vi "Main.vi"() -> ()   [LabVIEW 2020]
uses:
  <vilib>/Utility/config.llb/Read Key (String).vi
  <vilib>/Utility/file.llb/Write Delimited Spreadsheet (string).vi
  <vilib>/Utility/config.llb/NI_LVConfig.lvlib
panel:
  out "状态显示":bool=TRUE
  in  "开始测试":bool
  out "绝缘电阻采样测试":T1={"正极绝缘电阻"=0.0, "负极绝缘电阻"=0.0, "总判定"=TRUE}
  out "电流校准测试结果":T2={"表格控件"=[], "斜率"=0.0, "截距"=0.0, "判定"=TRUE}
  out "导通电阻":T3={"阻值"={"主保险"=0.0, "主正继电器"=0.0, "快充继电器"=0.0, "主负继电器"=0.0, "分流器"=0.0}, "判定"={"布尔"=TRUE, "布尔 2"=TRUE, "布尔 3"=TRUE, "布尔 4"=TRUE, "布尔 5"=TRUE}}
  out "Vact判定":bool=TRUE
  out "表格控件":string[][](table) caption="电压采样精度检测"
  out "短接快充":T4={"簇"={"Va"=0, "Vc"=0, "Vd"=0, "Vg"=0}, "判定"={"判定"=TRUE, "判定"=TRUE, "判定"=TRUE, "判定"=TRUE}}
  out "闭合主正快充":T4={"簇"={"Va"=0, "Vc"=0, "Vd"=0, "Vg"=0}, "判定"={"判定"=TRUE, "判定"=TRUE, "判定"=TRUE, "判定"=TRUE}}
  out "闭合主正":T4={"簇"={"Va"=0, "Vc"=0, "Vd"=0, "Vg"=0}, "判定"={"判定"=TRUE, "判定"=TRUE, "判定"=TRUE, "判定"=TRUE}}
  out "全部打开":T4={"簇"={"Va"=0, "Vc"=0, "Vd"=0, "Vg"=0}, "判定"={"判定"=TRUE, "判定"=TRUE, "判定"=TRUE, "判定"=TRUE}}
  out "预充电阻":dbl
  out "通断检测":T5={"粘连检测"={TRUE, TRUE, TRUE}, "导通检测"={"主保险"=0.0, "主正继电器"=0.0, "主负继电器"=0.0, "快充继电器"=0.0}, "簇"={TRUE, TRUE, TRUE, TRUE}}
  out "HVIL":T7={"占空比"=0, "频率/周期"=0, "软件版本号"=0, "频率判定"=TRUE, "占空比判定"=TRUE, "软件版本指示"=0} {"软件版本指示" items=["for 广汽新能源"=24015, "for 中航锂电"=25018]}
  out "CMC":cluster{"表格控件":string[][], "啊打发":bool}={"表格控件"=[], "啊打发"=TRUE}
  in  "停止":bool
  in  "value":string caption="序列号"
  # "F020电性能测试"
  # "47~53Ω"
  # "240~360kΩ"
  # "400~600kΩ"
  # "≤0.3"
  # "≤0.5"
  # "≤0.5"
  # "≤0.5"
  # "≤0.15"
  # "主正&预充"
  # "主负"
  # "快充"
  # "HVIL测试"
  # "Hz"
  # "判定：7~11Hz"
  # "判定：50±4%"
  # "%"
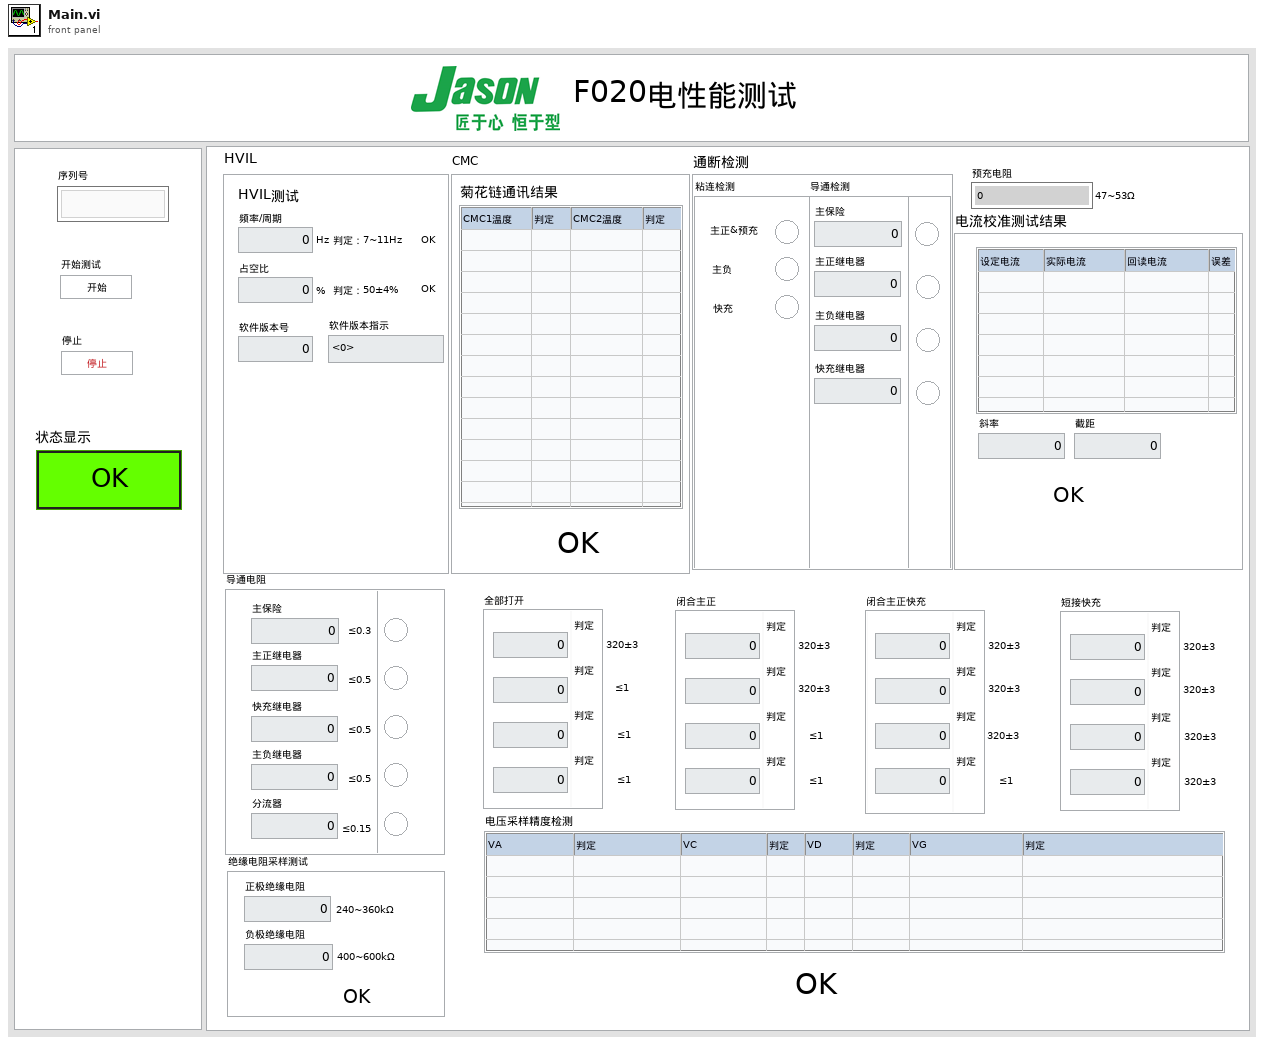
[diagram p1: front panel]
types:
  T1 = typedef "绝缘电阻测试.ctl" = cluster{"正极绝缘电阻":dbl, "负极绝缘电阻":dbl, "总判定":bool}
  T2 = typedef "电流校准测试.ctl" = cluster{"表格控件":string[][], "斜率":dbl, "截距":dbl, "判定":bool}
  T3 = typedef "导通电阻.ctl" = cluster{"阻值":cluster{"主保险":dbl, "主正继电器":dbl, "快充继电器":dbl, "主负继电器":dbl, "分流器":dbl}, "判定":cluster{"布尔":bool, "布尔 2":bool, "布尔 3":bool, "布尔 4":bool, "布尔 5":bool}}
  T4 = typedef "闭合主正.ctl" = cluster{"簇":cluster{"Va":u32, "Vc":u32, "Vd":u32, "Vg":u32}, "判定":cluster{"判定":bool, "判定":bool, "判定":bool, "判定":bool}}
  T5 = typedef "导通.ctl" = cluster{"粘连检测":cluster{bool, bool, bool}, "导通检测":cluster{"主保险":dbl, "主正继电器":dbl, "主负继电器":dbl, "快充继电器":dbl}, "簇":cluster{bool, bool, bool, bool}}
  T6 = typedef "软件版本指示.ctl" = u32
  T7 = cluster{"占空比":u32, "频率/周期":u32, "软件版本号":u32, "频率判定":bool, "占空比判定":bool, "软件版本指示":T6}
  T8 = typedef "状态机.ctl" = enum16{"Idle", "power on", "comm test", "conduct test", "resistance test", "Vact test", "insl test", "curr cal", "power off", "data log", "exit"}
  T9 = typedef "仪器地址输入.ctl" = cluster{"[0]":string, "[PLC]":string, "[IT6332B-1]":string, "[IT6332B-2]":string, "[2700-1]":string, "[2700-2]":string, "[TDK]":string, "[2410]":string}
  T10 = typedef "仪器实例.ctl" = cluster{"[0]":string, "[PLC]":refnum<k24>, "[IT6332B-1]":string, "[IT6332B-2]":string, "[2700-1]":string, "[2700-2]":string, "[TDK]":string, "[2410]":string}
  T11 = typedef "NI_LVConfig.lvlib/Config Data RefNum.ctl" = refnum<k1>
  T12 = cluster{"粘连判断[0]":bool, "粘连判断[1]":bool, "粘连判断[2]":bool}
  T13 = cluster{"导通值[0]":dbl, "导通值[1]":dbl, "导通值[2]":dbl, "导通值[3]":dbl}
  T14 = cluster{"导通判断[0]":bool, "导通判断[1]":bool, "导通判断[2]":bool, "导通判断[3]":bool}
  T15 = cluster{"导通电阻[0]":dbl, "导通电阻[1]":dbl, "导通电阻[2]":dbl, "导通电阻[3]":dbl, "导通电阻[4]":dbl}
  T16 = cluster{"x <= y?[0]":bool, "x <= y?[1]":bool, "x <= y?[2]":bool, "x <= y?[3]":bool, "x <= y?[4]":bool}
  T17 = cluster{"导通电阻":cluster{"导通电阻[0]":dbl, "导通电阻[1]":dbl, "导通电阻[2]":dbl, "导通电阻[3]":dbl, "导通电阻[4]":dbl}, "x <= y?":cluster{"x <= y?[0]":bool, "x <= y?[1]":bool, "x <= y?[2]":bool, "x <= y?[3]":bool, "x <= y?[4]":bool}}
  T18 = cluster{"布尔":bool, "布尔 2":bool, "布尔 3":bool, "布尔 4":bool, "布尔 5":bool}
  T19 = cluster{"主保险":dbl, "主正继电器":dbl, "快充继电器":dbl, "主负继电器":dbl, "分流器":dbl}
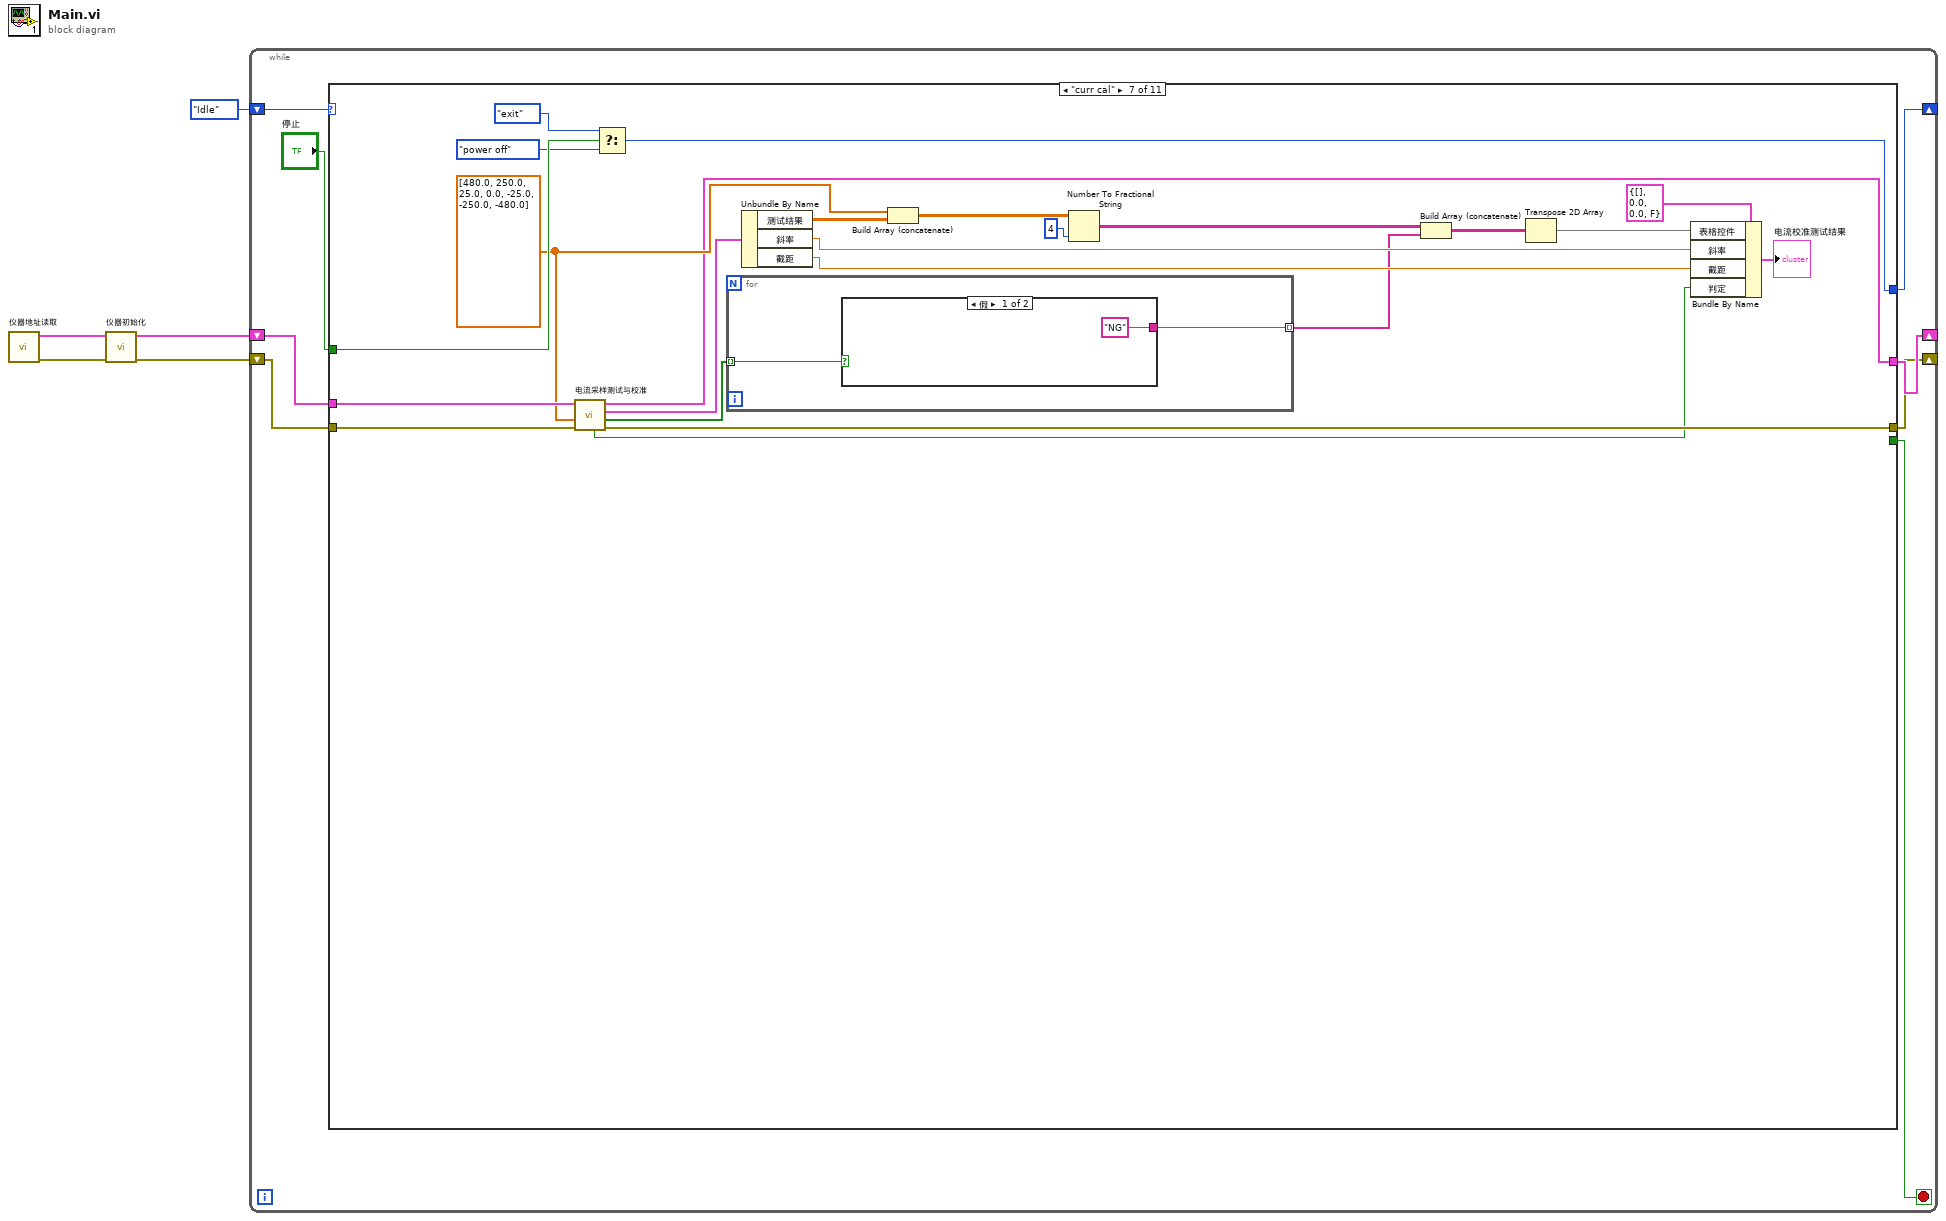
[diagram p0: block diagram]
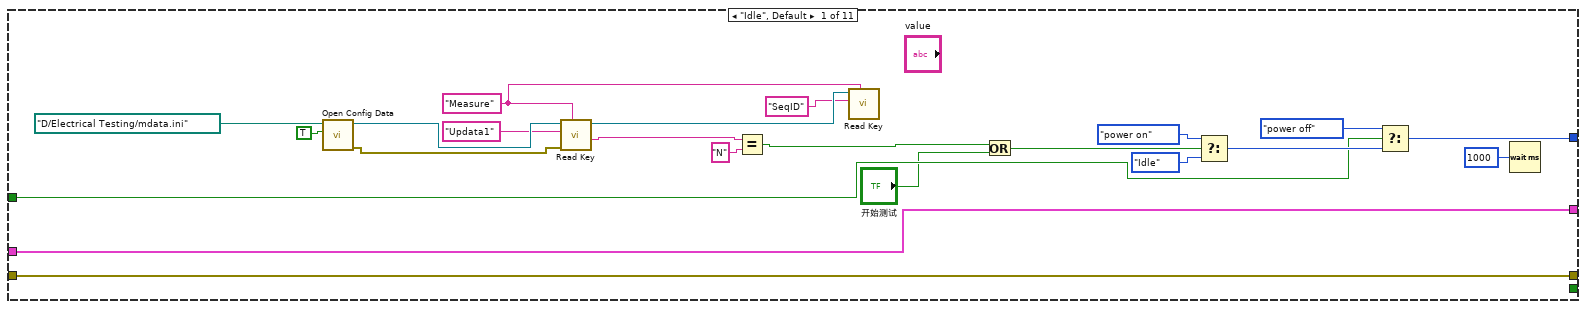
[diagram p2: hidden frame]
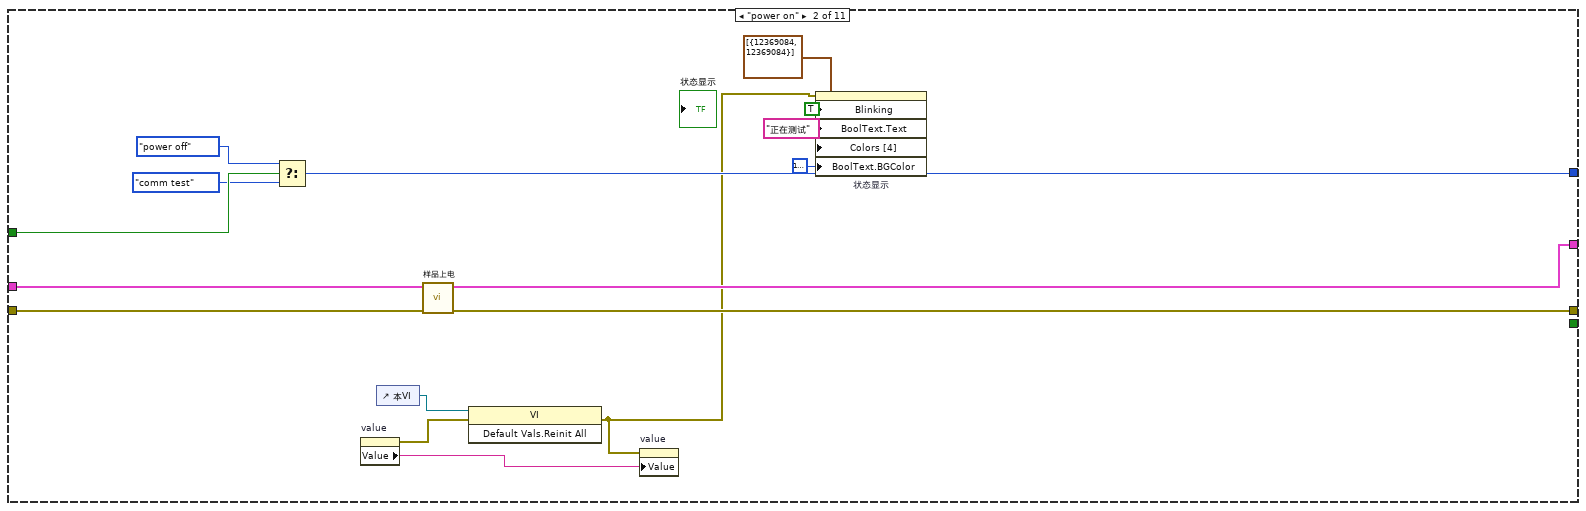
[diagram p3: hidden frame]
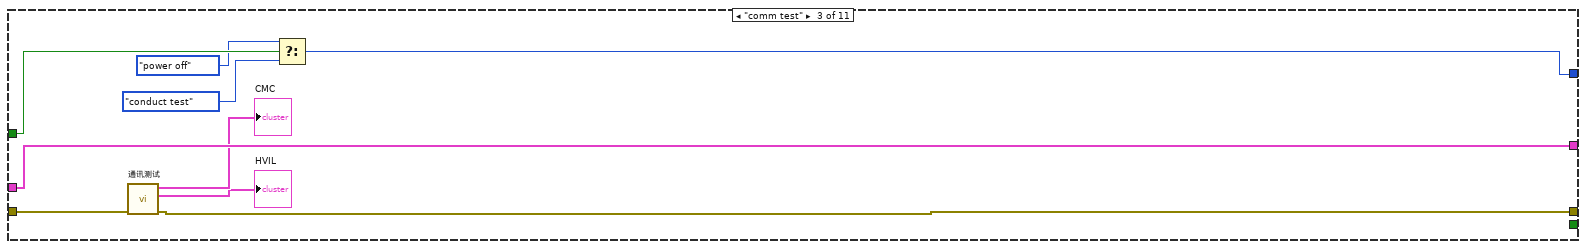
[diagram p4: hidden frame]
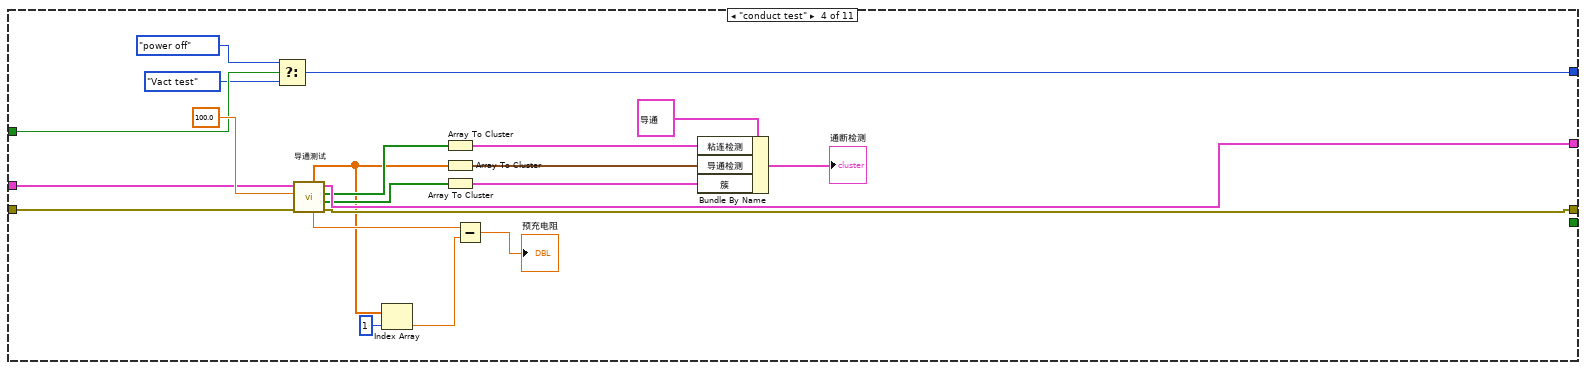
[diagram p5: hidden frame]
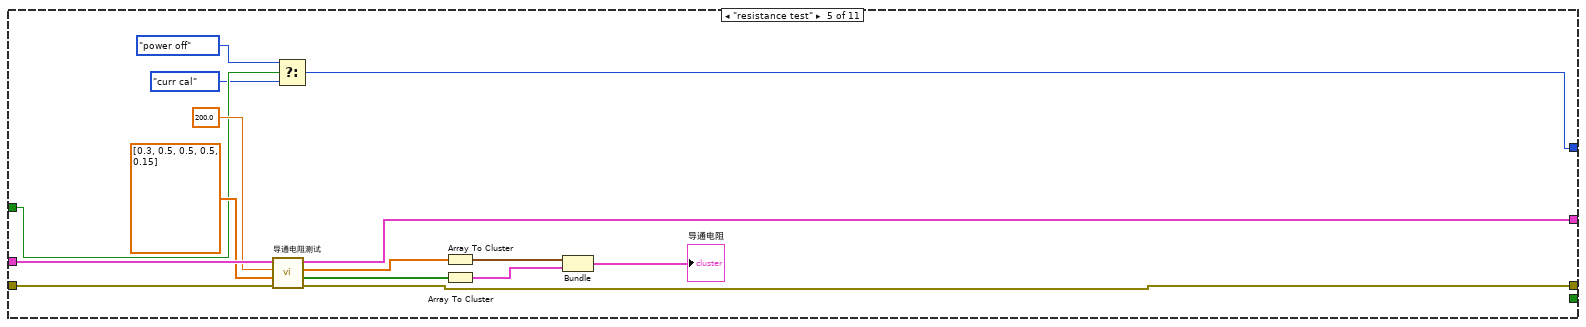
[diagram p6: hidden frame]
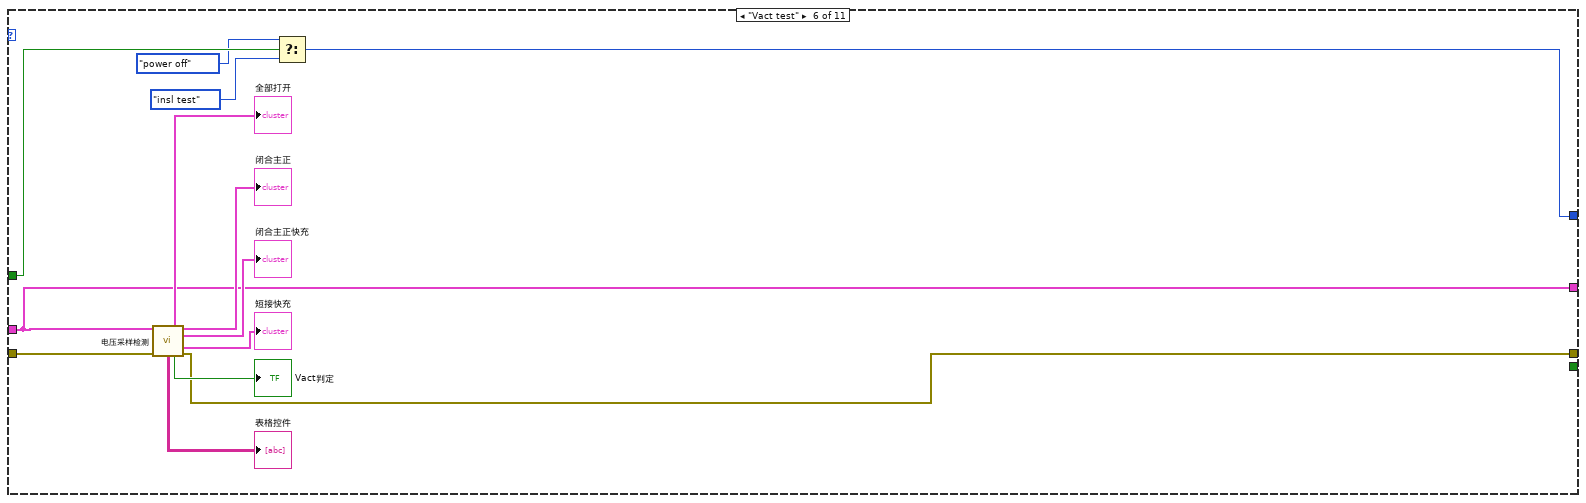
[diagram p7: hidden frame]
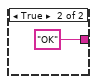
[diagram p8: hidden frame]
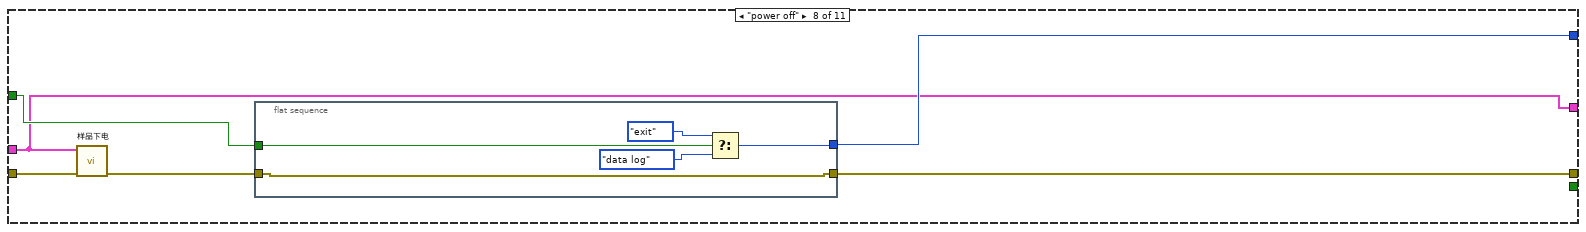
[diagram p9: hidden frame]
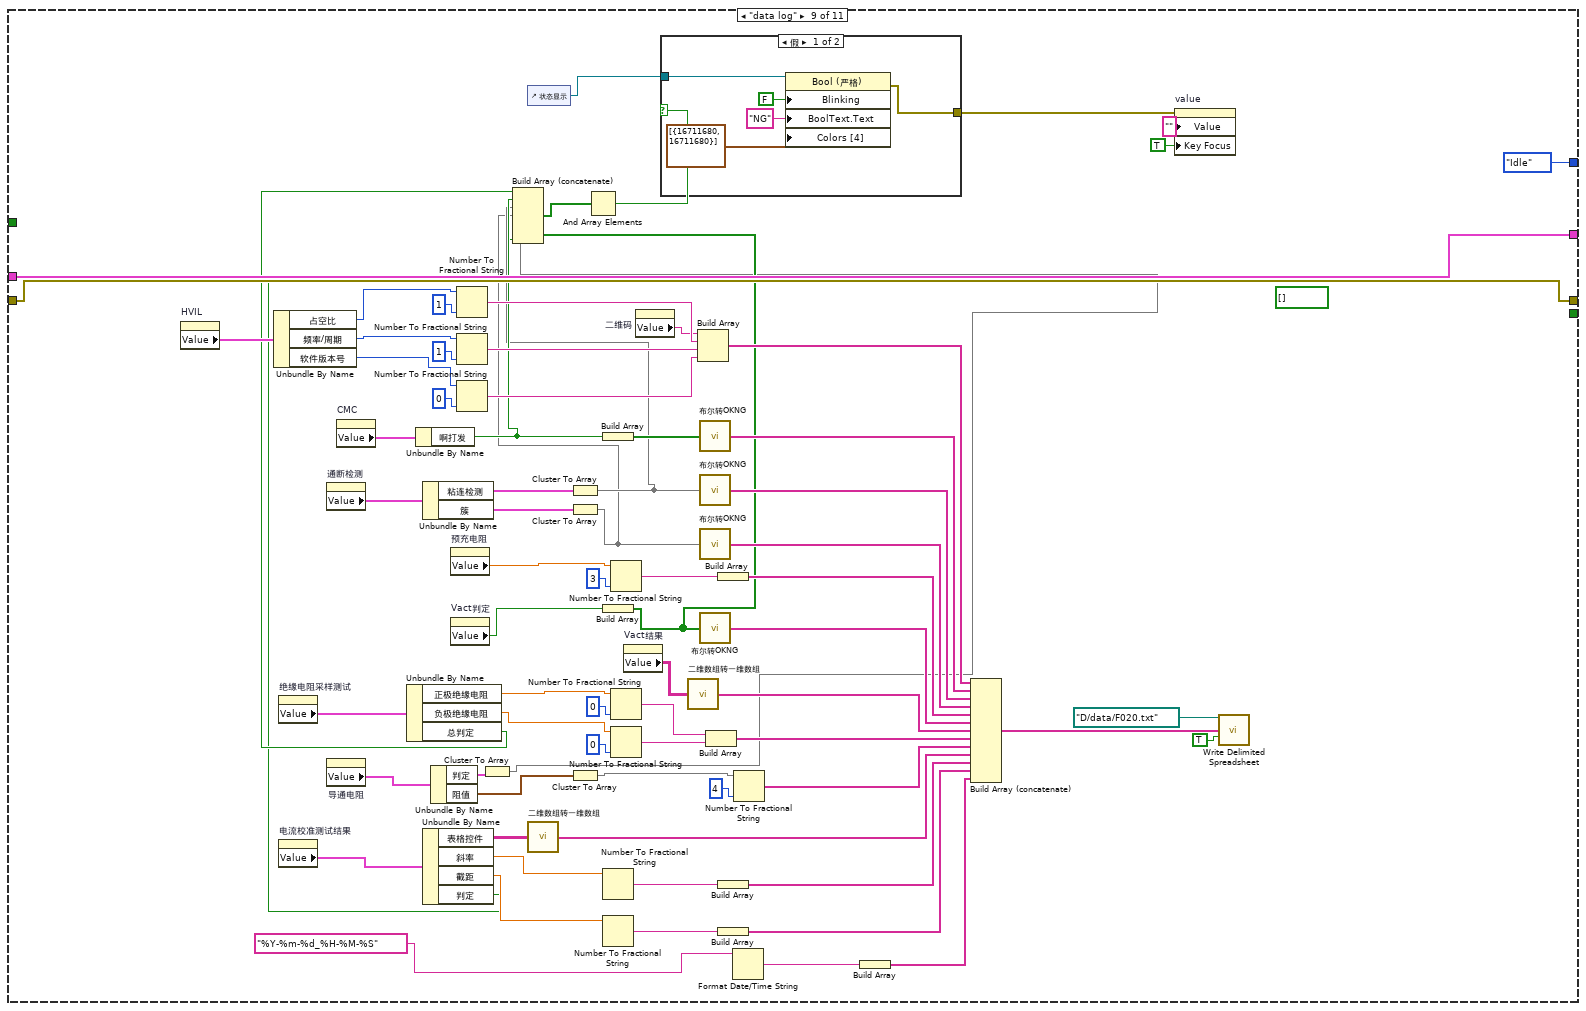
[diagram p10: hidden frame]
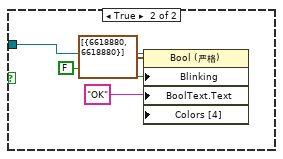
[diagram p11: hidden frame]
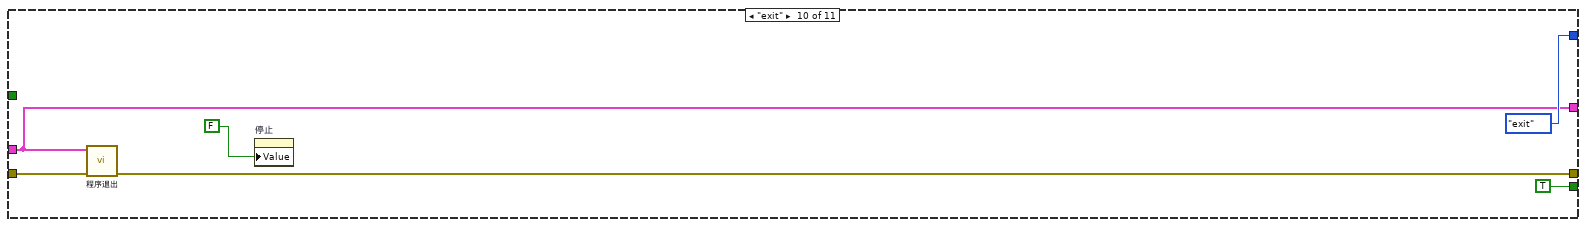
[diagram p12: hidden frame]
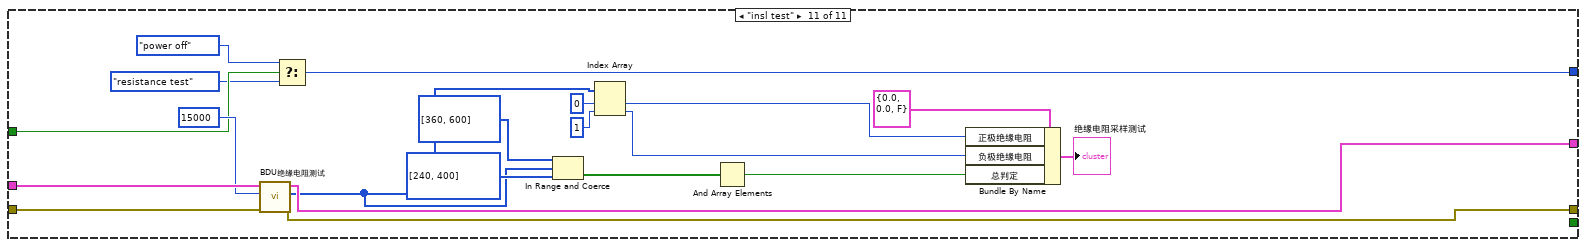
[diagram p13: hidden frame]
diagram:
  n1 = call "仪器地址读取.vi"() -> ("error out"=w5:errorcluster, "仪器地址"=w4:T9)  [unwired: 8 in]
  n2 = call "仪器初始化.vi"("错误输入（无错误）"=w5, "仪器地址"=w4) -> ("error out"=w1:errorcluster, "仪器实例 out"=w2:T10)  [unwired: 8 in]
  n3 = while {
    shift-right: [w13] -> _
    shift-left: 状态机."Idle" -> [w7]
    shift-right: [w9] -> _
    shift-left: w2 -> [w12]
    shift-right: [w8] -> _
    shift-left: w1 -> [w11]
    stop <- w6 stop-if-true
    n4 = case shown="\"curr cal\"" w7 {
      tunnel: [w24 w46 w55 w66 w82 w97 w118 w139 状态机."Idle" 状态机."exit" w247] -> w13
      tunnel: w12 -> [w18 w51 w59 w80 w96 w101 w117 w138 w220 w234 w255]
      tunnel: w11 -> [w17 w50 w60 w79 w92 w109 w115 w142 w163 w233 w253]
      tunnel: "停止" -> [w22 w47 w54 w67 w84 w100 w121 w140 _ _ w250]
      tunnel: [w18 w49 w59 w77 w93 w101 w114 w138 w220 w234 w251] -> w9
      tunnel: [w17 w48 w58 w78 w91 w102 w111 w137 w163 w232 w252] -> w8
      tunnel: [_ _ _ _ _ _ _ _ _ TRUE _] -> w6
      frame "Idle", Default {
        w29 = "Measure" ("section")
        n5 = call <vilib>:"Open Config Data.vi"("create file if necessary (T)"=TRUE, "configuration file path"=path "D:/Electrical Testing/mdata.ini") -> ("error out"=w33:errorcluster, "refnum"=w32:T11)  [unwired: 7 in, 1 out]
        n6 = call-poly <vilib>:"Read Key.vi"("section"=w29, "error in (no error)"=w33, "key"="Updata1", "refnum"=w32) -> ("value"=w27:string, "refnum out"=w30:T11)  [unwired: 4 in, 2 out]
        n7 = Equal?(x=w27, y="N") -> (x = y?=w16:bool)
        n8 = call-poly <vilib>:"Read Key.vi"("section"=w29, "key"="SeqID", "refnum"=w30) -> ()  [unwired: 5 in, 4 out]
        n9 = Or(x=w16, y="开始测试") -> (x .or. y?=w14:bool)
        n10 = Select(t=状态机."power on", s=w14, f=状态机."Idle") -> (s? t:f=w25:T8)
        n11 = Select(t=状态机."power off", s=w22, f=w25) -> (s? t:f=w24:T8)
        n12 = Wait (ms)(milliseconds to wait=u32 1000 ("等待时间（毫秒）")) -> ()  [unwired: 1 out]
      }
      frame "power on" {
        n13 = Select(t=状态机."power off", s=w47, f=状态机."comm test") -> (s? t:f=w46:T8)
        n14 = property on="value" class="Str"() -> (error out=w38:errorcluster, "Value"=w36:string)  [unwired: 2 in, 1 out]
        n15 = control-ref of="本VI"() -> (w43:refnum<vi>)
        n16 = call "样品上电.vi"("error in (no error)"=w50, "仪器实例 out"=w51) -> ("error out"=w48:errorcluster, "仪器实例 out 2"=w49:T10)  [unwired: 6 in]
        n17 = invoke class="VI" method="Default Vals.Reinit All"(reference=w43, error in=w38) -> (error out=w37:errorcluster)  [unwired: 1 in, 2 out]
        n18 = property on="value" class="Str"(error in=w37, "Value"=w36) -> ()  [unwired: 1 in, 2 out]
        n19 = property on="状态显示" class="Bool (严格)"(error in=w37, "Blinking"=TRUE ("闪烁"), "BoolText.Text"="正在测试" ("布尔文本.文本"), "Colors [4]"=cluster{u32, u32}[] [{12369084, 12369084}] ("颜色[4]"), "BoolText.BGColor"=u32 16777216 ("布尔文本.文本颜色:背景色")) -> ()  [unwired: 1 in, 2 out]
      }
      frame "comm test" {
        n20 = call "通讯测试.vi"("error in"=w60) -> ("CMC"=→"CMC":cluster{"表格控件":string[][], "啊打发":bool}, "HVIL"=→"HVIL":T7, "error out"=w58:errorcluster)  [unwired: 5 in]
        n21 = Select(t=状态机."power off", s=w54, f=状态机."conduct test") -> (s? t:f=w55:T8)
      }
      frame "conduct test" {
        n22 = Select(t=状态机."power off", s=w67, f=状态机."Vact test") -> (s? t:f=w66:T8)
        n23 = call "导通测试.vi"("error in (no error)"=w79, "导通阈值"=100.0, "仪器实例 in"=w80) -> ("error out"=w78:errorcluster, "导通判断"=w75:bool[], "粘连判断"=w76:bool[], "仪器实例 out"=w77:T10, "预充电阻"=w69:dbl, "导通值"=w63:dbl[])  [unwired: 3 in]
        n24 = Index Array(array=w63, index=1 ("索引")) -> (element=w61:dbl)
        n25 = Array To Cluster(array=w76) -> (cluster=w73:T12)
        n26 = Array To Cluster(array=w63) -> (cluster=w72:T13)
        n27 = Array To Cluster(array=w75) -> (cluster=w71:T14)
        n28 = Subtract(x=w69, y=w61) -> (x-y=→"预充电阻":dbl)
        n29 = Bundle By Name(cluster=T5 {"粘连检测"={FALSE, FALSE, FALSE}, "导通检测"={"主保险"=0.0, "主正继电器"=0.0, "主负继电器"=0.0, "快充继电器"=0.0}, "簇"={FALSE, FALSE, FALSE, FALSE}} ("通断检测"), "粘连检测"=w73, "导通检测"=w72, "簇"=w71) -> (→"通断检测":T5)
      }
      frame "resistance test" {
        n30 = call "导通电阻测试.vi"("error in (no error)"=w92, "接触电阻判断阈值"=dbl[] [0.3, 0.5, 0.5, 0.5, 0.15], "输入电流"=200.0, "仪器实例 in"=w96) -> ("error out"=w91:errorcluster, "x <= y?"=w90:bool[], "导通电阻"=w89:dbl[], "仪器实例 out"=w93:T10)  [unwired: 2 in]
        n31 = Select(t=状态机."power off", s=w84, f=状态机."curr cal") -> (s? t:f=w82:T8)
        n32 = Array To Cluster(array=w89) -> (cluster=w88:T15)
        n33 = Array To Cluster(array=w90) -> (cluster=w87:T16)
        n34 = Bundle("导通电阻"=w88, "x <= y?"=w87) -> (→"导通电阻":T17)  [unwired: 1 in]
      }
      frame "Vact test" {
        n35 = call "电压采样检测.vi"("仪器实例 in"=w101, "error in (no error)"=w109) -> ("全部打开"=→"全部打开":T4, "闭合主正"=→"闭合主正":T4, "闭合主正快充"=→"闭合主正快充":T4, "短接快充"=→"短接快充":T4, "表格控件"=→"表格控件":string[][], 14:→"Vact判定":bool, "error out"=w102:errorcluster)  [unwired: 7 in]
        n36 = Select(t=状态机."power off", s=w100, f=状态机."insl test") -> (s? t:f=w97:T8)
      }
      frame "curr cal" {
        w116 = dbl[] [480.0, 250.0, 25.0, 0.0, -25.0, -250.0, -480.0]
        n37 = call "电流采样测试与校准.vi"("仪器实例 in"=w117, 2:w116, "error in"=w115) -> ("总判定"=w110:bool, "仪器实例 out"=w114:T10, "测试结果"=w113:cluster{"测试结果":dbl[][], "斜率":dbl, "截距":dbl}, "判定数组"=w112:bool[], "error out"=w111:errorcluster)  [unwired: 3 in]
        n38 = Select(t=状态机."exit", s=w121, f=状态机."power off") -> (s? t:f=w118:T8)
        n39 = for {
          tunnel: w112 -> [w134] mode=indexing
          tunnel: [w133] -> w125 mode=indexing
          n40 = case shown="假" w134 {
            tunnel: ["NG" "OK"] -> w133
            frame False {
            }
            frame True {
            }
          }
        }
        n41 = Unbundle By Name(w113) -> ("测试结果"=w132:dbl[][], "斜率"=w129:dbl, "截距"=w128:dbl)
        n42 = Build Array (concatenate)(w116, w132) -> (w127:dbl[][])
        n43 = Number To Fractional String(number=w127, precision (6)=i16 4 ("精度(6)")) -> (F-format string=w126:string[][])  [unwired: 2 in]
        n44 = Build Array (concatenate)(w126, w125) -> (w124:string[][])
        n45 = Transpose 2D Array(2D array=w124) -> (transposed array=w123:string[][])
        n46 = Bundle By Name(cluster=T2 {"表格控件"=[], "斜率"=0.0, "截距"=0.0, "判定"=FALSE} ("校准测试结果"), "表格控件"=w123, "斜率"=w129, "截距"=w128, "判定"=w110) -> (→"电流校准测试结果":T2)
      }
      frame "power off" {
        n47 = call "样品下电.vi"("error in (no error)"=w142, "仪器实例 out"=w138) -> ("error out"=w141:errorcluster)  [unwired: 6 in, 1 out]
        n48 = flat-sequence {
          tunnel: w141 -> [w143]
          tunnel: w140 -> [w147]
          tunnel: [w146] -> w139
          tunnel: [w143] -> w137
          frame #0 {
            n49 = Select(t=状态机."exit", s=w147, f=状态机."data log") -> (s? t:f=w146:T8)
          }
        }
      }
      frame "data log" {
        (unwired) bool[] [] ("数组")
        n50 = property on="HVIL" class="Clust (严格)"() -> ("Value"=w217:T7)  [unwired: 2 in, 2 out]
        n51 = Unbundle By Name(w217) -> ("占空比"=w203:u32, "频率/周期"=w202:u32, "软件版本号"=w201:u32)
        n52 = property on="绝缘电阻采样测试" class="Clust (严格)"() -> ("Value"=w184:T1)  [unwired: 2 in, 2 out]
        n53 = property on="电流校准测试结果" class="Clust (严格)"() -> ("Value"=w213:T2)  [unwired: 2 in, 2 out]
        n54 = property on="通断检测" class="Clust (严格)"() -> ("Value"=w216:T5)  [unwired: 2 in, 2 out]
        n55 = property on="导通电阻" class="Clust (严格)"() -> ("Value"=w210:T3)  [unwired: 2 in, 2 out]
        n56 = property on="CMC" class="Clust (严格)"() -> ("Value"=w218:cluster{"表格控件":string[][], "啊打发":bool})  [unwired: 2 in, 2 out]
        n57 = Unbundle By Name(w184) -> ("正极绝缘电阻"=w182:dbl, "负极绝缘电阻"=w180:dbl, "总判定"=w157:bool)
        n58 = Unbundle By Name(w218) -> ("啊打发"=w161:bool)
        n59 = Unbundle By Name(w216) -> ("粘连检测"=w215:cluster{bool, bool, bool}, "簇"=w214:cluster{bool, bool, bool, bool})
        n60 = Unbundle By Name(w213) -> ("表格控件"=w212:string[][], "斜率"=w174:dbl, "截距"=w173:dbl, "判定"=w154:bool)
        n61 = Unbundle By Name(w210) -> ("判定"=w156:T18, "阻值"=w209:T19)
        n62 = property on="预充电阻" class="DigNum (严格)"() -> ("Value"=w195:dbl)  [unwired: 2 in, 2 out]
        n63 = property on="Vact判定" class="Bool (严格)"() -> ("Value"=w193:bool)  [unwired: 2 in, 2 out]
        n64 = Number To Fractional String(number=w203, precision (6)=i16 1 ("精度(6)")) -> (F-format string=w200:string)  [unwired: 2 in]
        n65 = Number To Fractional String(number=w202, precision (6)=i16 1 ("精度(6)")) -> (F-format string=w199:string)  [unwired: 2 in]
        n66 = Number To Fractional String(number=w201, precision (6)=i16 0 ("精度(6)")) -> (F-format string=w198:string)  [unwired: 2 in]
        n67 = Cluster To Array(cluster=w156) -> (array=w155:bool[])
        n68 = control-ref of="状态显示"() -> (w151:refnum<vi>)
        n69 = call "二维数组转一维数组.vi"("表格控件 2"=w212) -> ("数组"=w175:string[])
        n70 = Cluster To Array(cluster=w215) -> (array=w160:bool[])
        n71 = Cluster To Array(cluster=w214) -> (array=w159:bool[])
        n72 = Cluster To Array(cluster=w209) -> (array=w207:dbl[])
        n73 = Build Array(w161) -> (w196:bool[])
        n74 = Build Array(w193) -> (w158:bool[])
        n75 = Build Array (concatenate)(w157, w161, w160, w159, w158, w155, w154) -> (w153:bool[])
        n76 = And Array Elements(Boolean array=w153) -> (logical AND=w152:bool)
        n77 = Number To Fractional String(number=w174) -> (F-format string=w172:string)  [unwired: 3 in]
        n78 = Number To Fractional String(number=w173) -> (F-format string=w171:string)  [unwired: 3 in]
        n79 = Number To Fractional String(number=w195, precision (6)=i16 3 ("精度(6)")) -> (F-format string=w188:string)  [unwired: 2 in]
        n80 = Number To Fractional String(number=w182, precision (6)=i16 0 ("精度(6)")) -> (F-format string=w179:string)  [unwired: 2 in]
        n81 = Number To Fractional String(number=w180, precision (6)=i16 0 ("精度(6)")) -> (F-format string=w178:string)  [unwired: 2 in]
        n82 = property on="Vact结果" class="Tbl (严格)"() -> ("Value"=w211:string[][])  [unwired: 2 in, 2 out]
        n83 = property on="二维码" class="Str"() -> ("Value"=w197:string)  [unwired: 2 in, 2 out]
        n84 = case shown="假" w152 {
          tunnel: w151 -> [w223 w227]
          tunnel: [w221 _] -> w148
          frame False {
            n85 = property on="属性节点" class="Bool (严格)"(reference=w223, "Blinking"=FALSE ("闪烁"), "BoolText.Text"="NG" ("布尔文本.文本"), "Colors [4]"=cluster{u32, u32}[] [{16711680, 16711680}] ("颜色[4]")) -> (error out=w221:errorcluster)  [unwired: 1 in, 1 out]
          }
          frame True {
            n86 = property on="属性节点" class="Bool (严格)"(reference=w227, "Blinking"=FALSE ("闪烁"), "BoolText.Text"="OK" ("布尔文本.文本"), "Colors [4]"=cluster{u32, u32}[] [{6618880, 6618880}] ("颜色[4]")) -> ()  [unwired: 1 in, 2 out]
          }
        }
        n87 = call "二维数组转一维数组.vi"("表格控件 2"=w211) -> ("数组"=w185:string[])
        n88 = Build Array(w197, w200, w199, w198) -> (w192:string[])
        n89 = call "布尔转OKNG.vi"("数组"=w196) -> ("数组 out"=w191:string[])
        n90 = call "布尔转OKNG.vi"("数组"=w160) -> ("数组 out"=w190:string[])
        n91 = call "布尔转OKNG.vi"("数组"=w159) -> ("数组 out"=w189:string[])
        n92 = call "布尔转OKNG.vi"("数组"=w158) -> ("数组 out"=w186:string[])
        n93 = Build Array(w179, w178) -> (w177:string[])
        n94 = Build Array(w188) -> (w187:string[])
        n95 = Build Array(w172) -> (w170:string[])
        n96 = Build Array(w171) -> (w169:string[])
        n97 = Format Date/Time String(time format string (%c)="%Y-%m-%d_%H-%M-%S" ("时间格式字符串(%c)")) -> (date/time string=w165:string)  [unwired: 2 in]
        n98 = Number To Fractional String(number=w207, precision (6)=i16 4 ("精度(6)")) -> (F-format string=w176:string[])  [unwired: 2 in]
        n99 = Build Array(w165) -> (w164:string[])
        n100 = Build Array (concatenate)(w192, w191, w190, w189, w187, w186, w185, w177, w176, w175, w170, w169, w164) -> (w168:string[])
        n101 = property on="value" class="Str"(error in=w148, "Value"="" ("value"), "Key Focus"=TRUE ("键选中")) -> ()  [unwired: 1 in, 2 out]
        n102 = call-poly <vilib>:"Write Delimited Spreadsheet.vi"("file path (dialog if empty)"=path "D:/data/F020.txt", "1D data"=w168, "append to file? (new file:F)"=TRUE) -> ()  [unwired: 11 in, 2 out]
      }
      frame "exit" {
        n103 = call "程序退出.vi"("error in (no error)"=w233, "仪器实例 in"=w234) -> ("error out"=w232:errorcluster)  [unwired: 7 in]
        n104 = property on="停止" class="Bool (严格)"("Value"=FALSE ("停止")) -> ()  [unwired: 2 in, 2 out]
      }
      frame "insl test" {
        n105 = call "BDU绝缘电阻测试.vi"("error in (no error)"=w253, "等待时间（毫秒）"=u32 15000, "仪器实例 in"=w255) -> ("错误输出"=w252:errorcluster, "绝缘电阻"=w241:u16[], "仪器实例 out"=w251:T10)  [unwired: 6 in]
        n106 = Select(t=状态机."power off", s=w250, f=状态机."resistance test") -> (s? t:f=w247:T8)
        n107 = In Range and Coerce(upper limit=u16[] [360, 600] ("上限"), x=w241, lower limit=u16[] [240, 400] ("下限")) -> (In Range?=w244:bool[])  [unwired: 1 out]
        n108 = Index Array(array=w241, index #1=0 ("索引"), index #2=1 ("索引")) -> (element #1=w238:u16, element #2=w237:u16)
        n109 = And Array Elements(Boolean array=w244) -> (logical AND=w242:bool)
        n110 = Bundle By Name(cluster=T1 {"正极绝缘电阻"=0.0, "负极绝缘电阻"=0.0, "总判定"=FALSE} ("绝缘电阻采样测试"), "正极绝缘电阻"=w238, "负极绝缘电阻"=w237, "总判定"=w242) -> (→"绝缘电阻采样测试":T1)
      }
    }
  }
